vi "Process Secondary.vi"(11 "Ship in":refnum<class "Ship.lvclass">) -> (2 "New Elements":refnum<class "Element.lvclass">[](array[class]), 3 "Ship out":refnum<class "Ship.lvclass">)   [LabVIEW 2021, in "Ship.lvclass"]
uses:
  Ship.lvclass
  Element/Element.lvclass
  Ship.lvclass/Ship.ctl
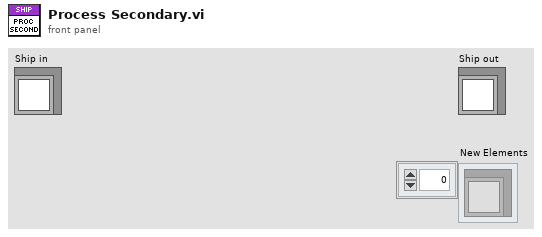
[diagram p1: front panel]
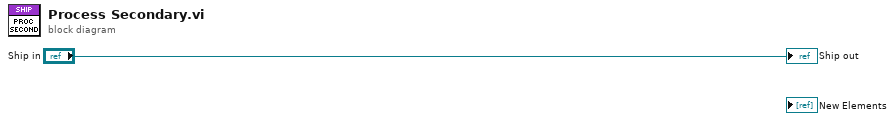
[diagram p0: block diagram]
diagram:
  "Ship out" <- "Ship in"
